vi "Wind Farm #1.vi"(8 "error in (no error)":errorcluster) -> (0 "error out":errorcluster)   [LabVIEW 2011]
doc: "This is one of 4 potential implementations for the Wind Farm Requirements. Specifically note how the wind turbine information is displayed. Also note how the main VI communicates back and forth to the wind turbine. What does that pipeline look like? Finally note the mechanism for stopping the wind turbine.\n\nAAL 9/09"
uses:
  Controls/File Type.ctl
  Controls/Stop FGV Commands.ctl
  Shared/QDMH Poly VIs/QDMH POLY Enqueue String.vi
panel:
  in  "File Type":T1 caption="File Type (Read When Turbine is Added)"
  out "Wind Turbine Speed":dbl=15.0
  in  "Set Wind Speed":bool
  in  "Wind Speed":dbl=15.0
  in  "Wind Turbine Selection":u16(ring)
  in  "Queue Name":string
  in  "Add Wind Turbine":bool
  in  "Save Data":bool
  out "Message Display":string
  in  "Exit":bool
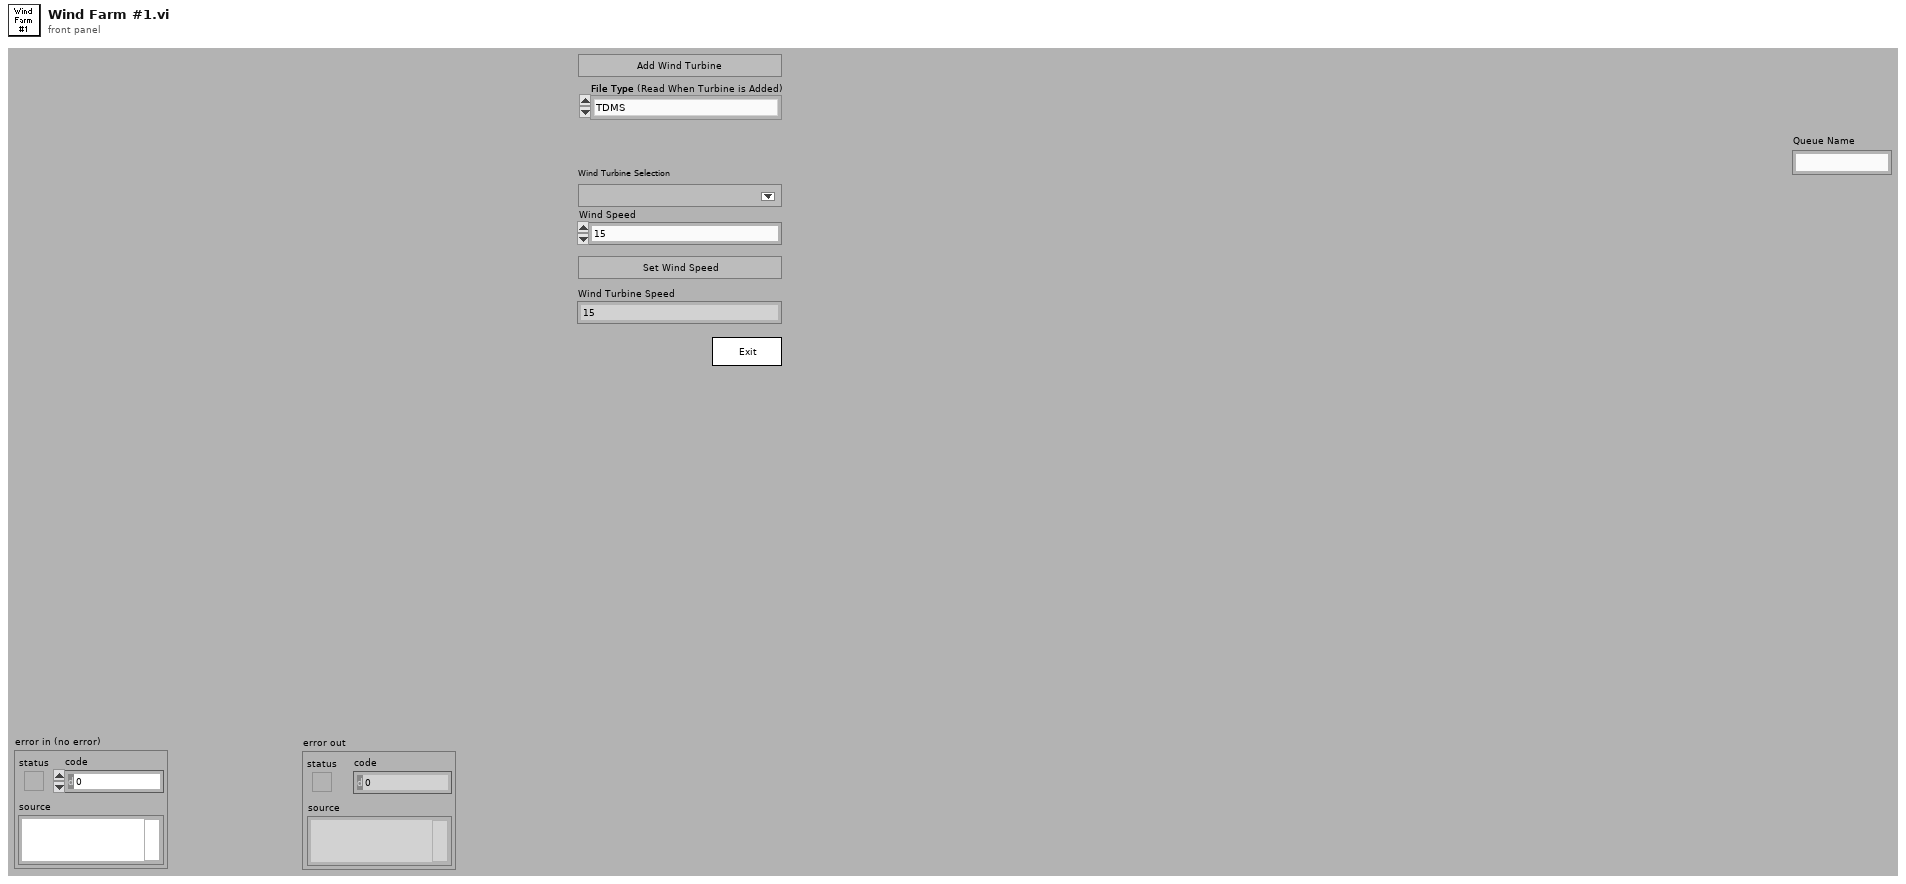
[diagram p1: front panel]
types:
  T1 = typedef "File Type.ctl" = enum16{"TDMS", "TXT"}
  T2 = cluster{"Operator Name":string, "Current VI's Path":path, "Main Directory":path, "Y Data":dbl[], "Ini Path":path, "Model":string, " VIT References":refnum<vi>[], "VIT Current":refnum<vi>, "VIT Path":path, "VIT Item Names ":string[], "Wind Speed":dbl, "Windmill Selection":i32, "Turbine Speed":dbl}
  T3 = typedef "Stop FGV Commands.ctl" = enum16{"Write", "Read", "Reset"}
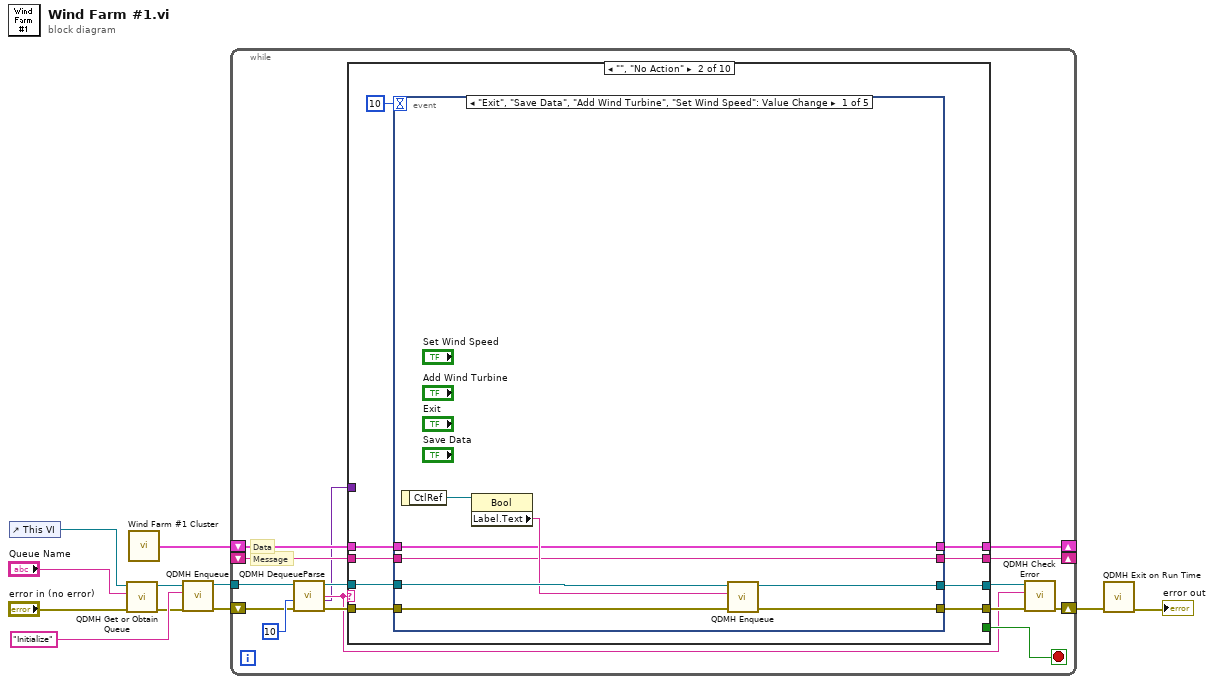
[diagram p0: block diagram]
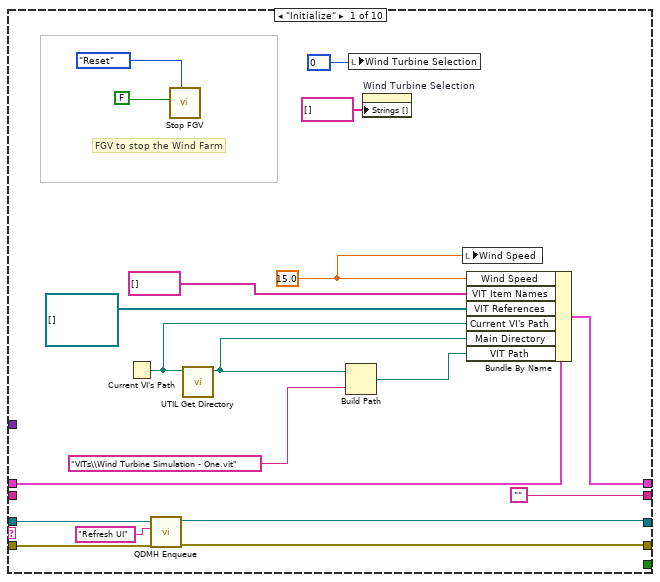
[diagram p2: hidden frame]
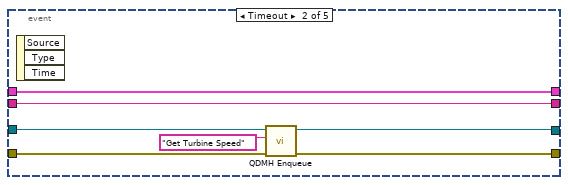
[diagram p3: hidden frame]
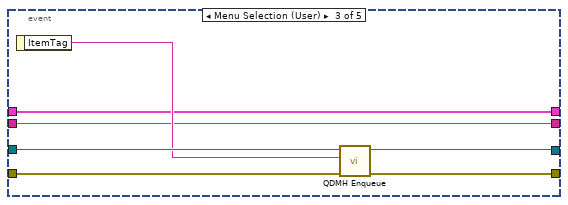
[diagram p4: hidden frame]
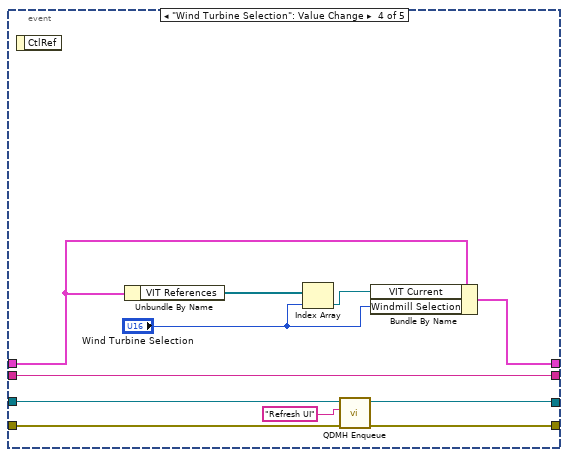
[diagram p5: hidden frame]
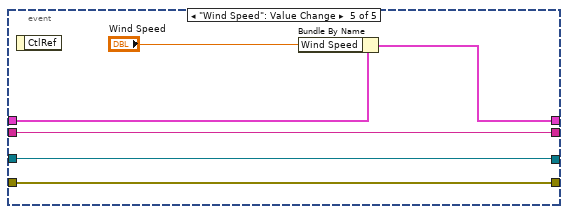
[diagram p6: hidden frame]
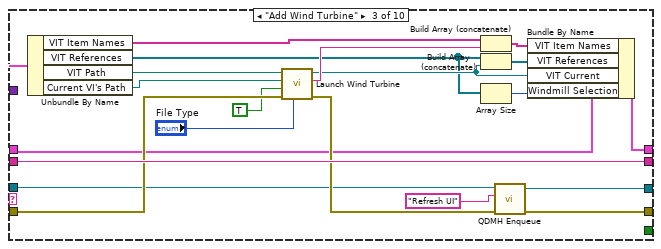
[diagram p7: hidden frame]
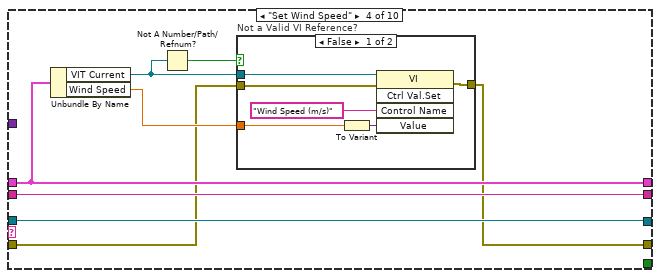
[diagram p8: hidden frame]
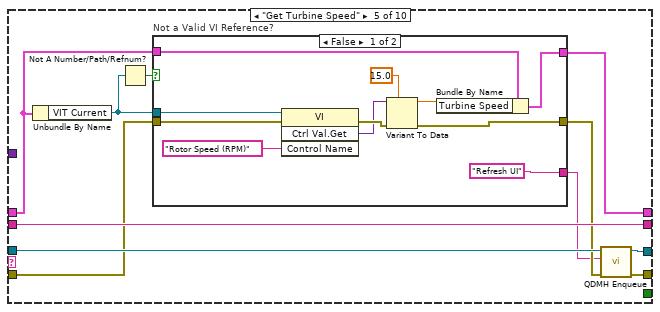
[diagram p10: hidden frame]
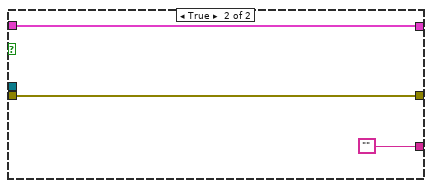
[diagram p11: hidden frame]
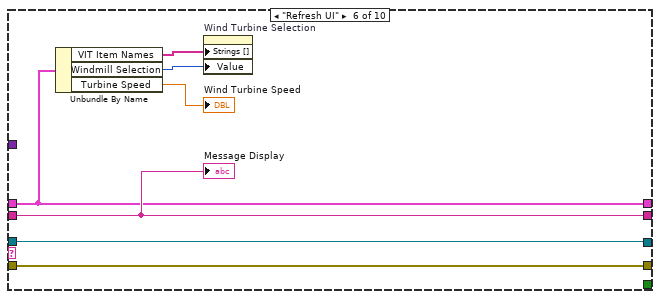
[diagram p12: hidden frame]
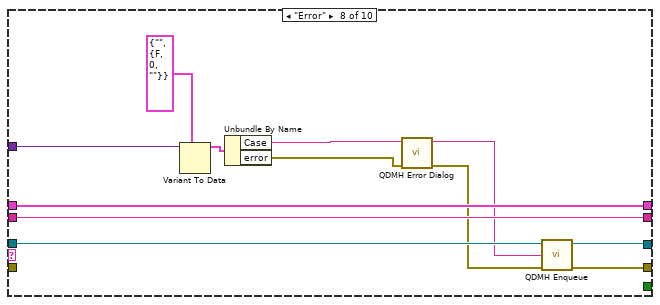
[diagram p14: hidden frame]
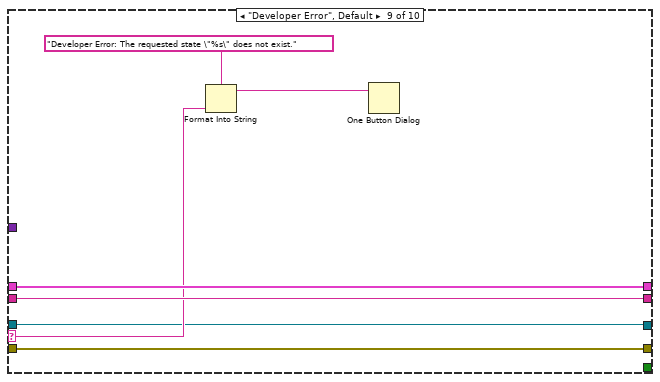
[diagram p15: hidden frame]
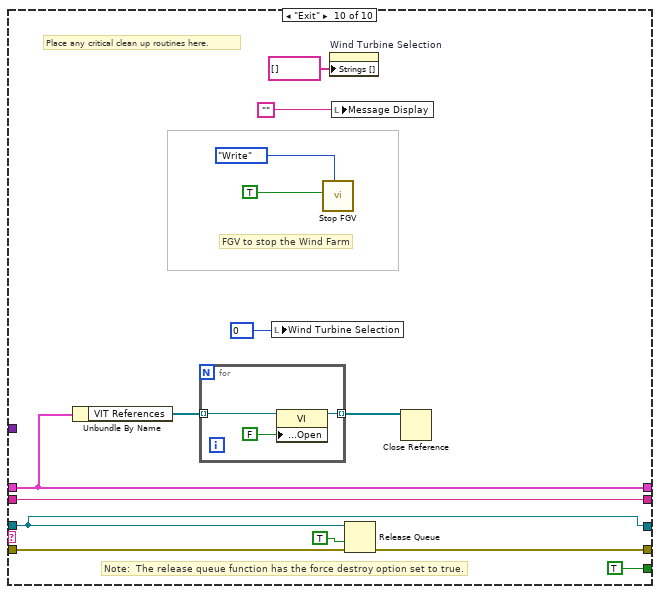
[diagram p16: hidden frame]
diagram:
  n1 = control-ref of="This VI"() -> (w1:refnum<vi>)
  n2 = call "QDMH Get or Obtain Queue.vi"("error in (no error)"="error in (no error)", "Queue Name"="Queue Name", "VI Refnum"=w1) -> ("error out"=w7:errorcluster, "queue out"=w10:refnum<queue>)  [unwired: 7 out]
  n3 = call "Wind Farm #1 Cluster.vi"() -> ("Cluster"=w3:T2)
  n4 = call-poly "QDMH Enqueue.vi"("error in (no error)"=w7, "State"="Initialize" ("element"), "queue"=w10) -> ("error out"=w8:errorcluster, "queue out"=w11:refnum<queue>)  [unwired: 7 out]
  n5 = while {
    tunnel: w11 -> [w21]
    shift-left: w3 -> [w22]
    shift-right: [w23] -> _
    shift-left: _ -> [w24]
    shift-right: [w25] -> _
    shift-right: [w15] -> w5
    shift-left: w8 -> [w17]
    stop <- w26 stop-if-true
    # "Data"
    # "Message"
    n6 = call "QDMH DequeueParse.vi"("error in (no error)"=w17, "Timeout"=10 ("ms timeout (-1)"), "queue"=w21) -> ("error out"=w18:errorcluster, "Variant Data"=w12:variant, "State"=w13:string, "queue out"=w19:refnum<queue>)  [unwired: 5 out]
    n7 = case shown="\"\", \"No Action\"" w13 {
      selector: w13 -> [_ _ _ _ _ _ _ _ w180 _]
      tunnel: w19 -> [w42 w54 w102 w120 w136 w157 w161 w174 w177 w194]
      tunnel: [_ _ _ _ _ _ _ _ _ TRUE] -> w26
      tunnel: ["" w47 w113 w121 w139 w159 w164 w176 w183 w196] -> w25
      tunnel: w24 -> [_ w48 w113 w121 w139 w159 w164 w176 w183 w196]
      tunnel: [w44 w49 w99 w119 w137 w158 w163 w175 w182 w190] -> w23
      tunnel: w22 -> [w45 w50 w100 w119 w138 w158 w163 w175 w182 w190]
      tunnel: w18 -> [w41 w53 w110 w115 w133 w160 w162 _ w179 w193]
      tunnel: [w40 w52 w104 w114 w135 w160 w162 w173 w179 w192] -> w16
      tunnel: [w28 w46 w103 w120 w134 w157 w161 w172 w177 w194] -> w14
      tunnel: w12 -> [_ _ _ _ _ _ _ w167 _ _]
      frame "Initialize" {
        w30 = u16 0 items=[""] ("1 Windmill Selection")
        w29 = 15.0 ("1 Wind Speed")
        # "FGV to stop the Wind Farm"
        n8 = Current VI's Path() -> (path=w38:path)
        n9 = call-poly "QDMH Enqueue.vi"("error in (no error)"=w41, "State"="Refresh UI" ("element"), "queue"=w42) -> ("error out"=w40:errorcluster, "queue out"=w28:refnum<queue>)  [unwired: 7 out]
        n10 = call "Stop FGV.vi"("Command"=Stop_FGV_Commands."Reset", "Stop?"=FALSE) -> ()  [unwired: 2 in, 8 out]
        n11 = call "UTIL Get Directory.vi"("Path In"=w38) -> ("Directory Out"=w37:path)  [unwired: 1 in, 9 out]
        n12 = Build Path(base path=w37, name or relative path="VITs\\Wind Turbine Simulation - One.vit") -> (appended path=w36:path)
        n13 = local write "Wind Turbine Selection"(w30) -> ()
        n14 = property on="Wind Turbine Selection" class="Ring (strict)"("Strings []"=string[] []) -> ()  [unwired: 2 in, 2 out]
        n15 = local write "Wind Speed"(w29) -> ()
        n16 = Bundle By Name(cluster=w45, "Wind Speed"=w29, "VIT Item Names"=string[] [] ("1 VIT Item Names"), "VIT References"=refnum<vi>[] [], "Current VI's Path"=w38, "Main Directory"=w37, "VIT Path"=w36) -> (w44:T2)
      }
      frame "", "No Action" {
        n17 = event shown="[0] \"Exit\", \"Save Data\", \"Add Wind Turbine\", \"Set Wind Speed\": Value Change" {
          selector: _ -> [_ _ _ _ _]
          dyn-events: _ -> [_ _ _ _ _]
          timeout: 10 -> [_ _ _ _ _]
          tunnel: w54 -> [w61 w67 w76 w87 w89]
          tunnel: [w60 w65 w74 w85 w88] -> w52
          tunnel: w53 -> [w59 w66 w75 w86 w88]
          tunnel: w50 -> [w55 w69 w72 w79 w92]
          tunnel: [w55 w69 w72 w78 w91] -> w49
          tunnel: w48 -> [w57 w68 w71 w84 w93]
          tunnel: [w57 w68 w71 w84 w93] -> w47
          tunnel: [w56 w64 w70 w83 w89] -> w46
          event "Exit", "Save Data", "Add Wind Turbine", "Set Wind Speed": Value Change {
            n18 = event-data() -> ("CtlRef"=w62:refnum<vi>)  [unwired: 1 out]
            n19 = property class="Bool"(reference=w62) -> ("Label.Text"=w58:string)  [unwired: 1 in, 2 out]
            n20 = call-poly "QDMH Enqueue.vi"("error in (no error)"=w59, "State"=w58, "queue"=w61) -> ("error out"=w60:errorcluster, "queue out"=w56:refnum<queue>)  [unwired: 7 out]
          }
          event Timeout {
            n21 = event-data() -> ()  [unwired: 4 out]
            n22 = call-poly "QDMH Enqueue.vi"("error in (no error)"=w66, "State"="Get Turbine Speed", "queue"=w67) -> ("error out"=w65:errorcluster, "queue out"=w64:refnum<queue>)  [unwired: 7 out]
          }
          event Menu Selection (User) {
            n23 = event-data() -> ("ItemTag"=w73:string)  [unwired: 1 out]
            n24 = call-poly "QDMH Enqueue.vi"("error in (no error)"=w75, "State"=w73, "queue"=w76) -> ("error out"=w74:errorcluster, "queue out"=w70:refnum<queue>)  [unwired: 7 out]
          }
          event "Wind Turbine Selection": Value Change {
            n25 = event-data() -> ()  [unwired: 2 out]
            n26 = Unbundle By Name(w79) -> ("VIT References"=w81:refnum<vi>[])
            n27 = Index Array(array=w81, index="Wind Turbine Selection") -> (element=w80:refnum<vi>)
            n28 = call-poly "QDMH Enqueue.vi"("error in (no error)"=w86, "State"="Refresh UI" ("element"), "queue"=w87) -> ("error out"=w85:errorcluster, "queue out"=w83:refnum<queue>)  [unwired: 7 out]
            n29 = Bundle By Name(cluster=w79, "VIT Current"=w80, "Windmill Selection"="Wind Turbine Selection") -> (w78:T2)
          }
          event "Wind Speed": Value Change {
            n30 = event-data() -> ()  [unwired: 2 out]
            n31 = Bundle By Name(cluster=w92, "Wind Speed"="Wind Speed") -> (w91:T2)
          }
        }
      }
      frame "Add Wind Turbine" {
        n32 = Unbundle By Name(w100) -> ("VIT Item Names"=w109:string[], "VIT References"=w98:refnum<vi>[], "VIT Path"=w112:path, "Current VI's Path"=w96:path)
        n33 = call "Launch Wind Turbine.vi"("File Type"="File Type", "error in"=w110, "Front Panel Open?"=TRUE, "Calling VI Path"=w96, "VIT Path"=w112) -> ("error out"=w105:errorcluster, "Name"=w108:string, "vi reference"=w106:refnum<vi>)  [unwired: 4 in]
        n34 = Build Array (concatenate)(w109, w108) -> (w107:string[])
        n35 = Build Array (concatenate)(w98, w106) -> (w111:refnum<vi>[])
        n36 = Array Size(array=w98) -> (size(s)=w97:i32)
        n37 = call-poly "QDMH Enqueue.vi"("error in (no error)"=w105, "State"="Refresh UI" ("element"), "queue"=w102) -> ("error out"=w104:errorcluster, "queue out"=w103:refnum<queue>)  [unwired: 7 out]
        n38 = Bundle By Name(cluster=w100, "VIT Item Names"=w107, "VIT References"=w111, "VIT Current"=w106, "Windmill Selection"=w97) -> (w99:T2)
      }
      frame "Set Wind Speed" {
        n39 = Unbundle By Name(w119) -> ("VIT Current"=w116:refnum<vi>, "Wind Speed"=w118:dbl)
        n40 = Not A Number/Path/Refnum?(number/path/refnum=w116) -> (NaN/Path/Refnum?=w117:bool)
        n41 = case "Not a Valid VI Reference?" shown="False" w117 {
          tunnel: w116 -> [w127 _]
          tunnel: w118 -> [w125 _]
          tunnel: w115 -> [w123 w128]
          tunnel: [w122 w128] -> w114
          frame False {
            n42 = To Variant(anything=w125) -> (Variant=w124:variant)
            n43 = invoke class="VI" method="Ctrl Val.Set"(reference=w127, error in=w123, "Control Name"="Wind Speed (m/s)", "Value"=w124) -> (error out=w122:errorcluster)  [unwired: 1 in, 4 out]
          }
          frame True {
          }
        }
      }
      frame "Get Turbine Speed" {
        n44 = Unbundle By Name(w138) -> ("VIT Current"=w130:refnum<vi>)
        n45 = Not A Number/Path/Refnum?(number/path/refnum=w130) -> (NaN/Path/Refnum?=w129:bool)
        n46 = case "Not a Valid VI Reference?" shown="False" w129 {
          tunnel: w130 -> [w150 _]
          tunnel: w138 -> [w148 w153]
          tunnel: [w147 w153] -> w137
          tunnel: w133 -> [w142 w152]
          tunnel: [w141 w152] -> w132
          tunnel: ["Refresh UI" ("State") ""] -> w131
          frame False {
            n47 = invoke class="VI" method="Ctrl Val.Get"(reference=w150, error in=w142, "Control Name"="Rotor Speed (RPM)") -> (error out=w146:errorcluster, "Get Control Value Variant"=w145:variant)  [unwired: 1 in, 2 out]
            n48 = Variant To Data(error in=w146, type=15.0 ("Wind Turbine Speed"), Variant=w145) -> (data=w143:dbl, error out=w141:errorcluster)
            n49 = Bundle By Name(cluster=w148, "Turbine Speed"=w143) -> (w147:T2)
          }
          frame True {
          }
        }
        n50 = call-poly "QDMH Enqueue.vi"("error in (no error)"=w132, "State"=w131, "queue"=w136) -> ("error out"=w135:errorcluster, "queue out"=w134:refnum<queue>)  [unwired: 7 out]
      }
      frame "Refresh UI" {
        n51 = Unbundle By Name(w158) -> ("VIT Item Names"=w156:string[], "Windmill Selection"=w155:i32, "Turbine Speed"=→"Wind Turbine Speed":dbl)
        n52 = property on="Wind Turbine Selection" class="Ring (strict)"("Strings []"=w156, "Value"=w155) -> ()  [unwired: 2 in, 2 out]
        "Message Display" <- w159
      }
      frame "<add states as needed>" {
        # "Duplicate this state for any additional states that you add."
      }
      frame "Error" {
        n53 = Variant To Data(type=cluster{"Case":string, "error":errorcluster} {"Case"="", "error"={"status"=FALSE, "code"=0, "source"=""}} ("QDSM Element"), Variant=w167) -> (data=w170:cluster{"Case":string, "error":errorcluster})  [unwired: 1 in, 1 out]
        n54 = Unbundle By Name(w170) -> ("Case"=w169:string, "error"=w168:errorcluster)
        n55 = call "QDMH Error Dialog.vi"("error"=w168, "Case Error Occured"=w169) -> ("error out (no error)"=w165:errorcluster, "Case to Execute"=w166:string)  [unwired: 8 out]
        n56 = call-poly "QDMH Enqueue.vi"("error in (no error)"=w165, "State"=w166, "queue"=w174) -> ("error out"=w173:errorcluster, "queue out"=w172:refnum<queue>)  [unwired: 7 out]
      }
      frame "Developer Error", Default {
        n57 = Format Into String(format string="Developer Error: The requested state \"%s\" does not exist." ("message"), w180) -> (resulting string=w178:string)  [unwired: 2 in, 1 out]
        n58 = One Button Dialog(message=w178) -> ()  [unwired: 2 out]
      }
      frame "Exit" {
        w185 = u16 0 items=[""] ("1 Windmill Selection")
        # "FGV to stop the Wind Farm"
        # "Note:  The release queue function has the force destroy option set to true."
        # "Place any critical clean up routines here."
        n59 = Unbundle By Name(w190) -> ("VIT References"=w187:refnum<vi>[])
        n60 = for {
          tunnel: w187 -> [w200] mode=indexing
          tunnel: [w198] -> w186 mode=indexing
          n61 = property class="VI"(reference=w200, "Front Panel.Open"=FALSE ("Front Panel Window:Open")) -> (reference out=w198:refnum<vi>)  [unwired: 1 in, 1 out]
        }
        n62 = local write "Wind Turbine Selection"(w185) -> ()
        n63 = call "Stop FGV.vi"("Command"=Stop_FGV_Commands."Write", "Stop?"=TRUE) -> ()  [unwired: 2 in, 8 out]
        n64 = property on="Wind Turbine Selection" class="Ring (strict)"("Strings []"=string[] []) -> ()  [unwired: 2 in, 2 out]
        n65 = local write "Message Display"("") -> ()
        n66 = Release Queue(queue=w194, force destroy? (F)=TRUE, error in (no error)=w193) -> (error out=w192:errorcluster)  [unwired: 2 out]
        n67 = Close Reference(reference=w186) -> ()  [unwired: 1 in, 1 out]
      }
    }
    n68 = call "QDMH Check Error.vi"("error in (no error)"=w16, "Case"=w13, "queue"=w14) -> ("error out"=w15:errorcluster)  [unwired: 1 in, 7 out]
  }
  n69 = call "QDMH Exit on Run Time.vi"("error in (no error)"=w5) -> ("error out"=→"error out":errorcluster)  [unwired: 10 out]
